vi "Cheak File.vi"(6 "Station ID":string) -> (0 "true":bool)   [LabVIEW 2017]
uses:
  Ctrls/PathChoose.ctl
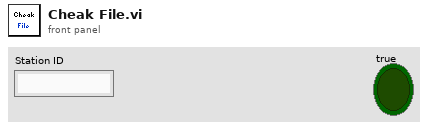
[diagram p1: front panel]
types:
  T1 = typedef "PathChoose.ctl" = enum16{"OperatorLog", "AutoRunLog", "AlmLog", "TestData", "AllTestData", "backup_nvm", "backup_before_flashing"}
  T2 = enum16{"open", "replace", "create", "open or create", "replace or create", "replace or create with confirmation"}
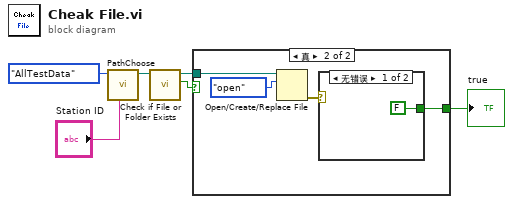
[diagram p0: block diagram]
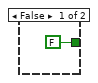
[diagram p2: hidden frame]
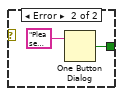
[diagram p3: hidden frame]
diagram:
  n1 = call "PathChoose.vi"("csv Name"="Station ID", 11:PathChoose."AllTestData") -> ("Path_Out"=w2:path)  [unwired: 9 in]
  n2 = call <vilib>:"Check if File or Folder Exists.vi"("path"=w2) -> ("file or folder exists?"=w4:bool, "dup path"=w5:path)  [unwired: 8 in, 1 out]
  n3 = case shown="真" w4 {
    tunnel: w5 -> [_ w10]
    tunnel: [FALSE ("true") w8] -> w3
    frame False {
    }
    frame True {
      n4 = Open/Create/Replace File(file path (use dialog)=w10, operation (0:open)=T2."open") -> (error out=w9:errorcluster)  [unwired: 4 in, 2 out]
      n5 = case shown="无错误" w9 {
        tunnel: [FALSE ("true") w13] -> w8
        frame No Error {
        }
        frame Error {
          n6 = One Button Dialog(message="Please Close The TsetData!") -> (true=w13:bool)  [unwired: 1 in]
        }
      }
    }
  }
  "true" <- w3
